vi "FormCalibra6.vi"() -> ()   [LabVIEW 2014]
uses:
  testMachine.ctl
  mainMachine.ctl
  <vilib>/Analysis/baseanly.llb/Mean (DBL).vi
  <vilib>/express/express shared/transition.llb/Dynamic To Waveform Array.vi
  <vilib>/express/express signal manip/GetorSetDDTAttributes/Set DDT Attributes/SetT0.vi
  <vilib>/express/express shared/transition.llb/Waveform Array To Dynamic.vi
  <vilib>/measure/mamon.llb/Trigger Detection for 1 Channel.vi
  <vilib>/express/express signal manip/GetorSetDDTAttributes/Set DDT Attributes/Set DDT Properties.xnode
  <vilib>/Analysis/NI_AALBase.lvlib
  <resource>/objmgr/daqmx.rc
  <vilib>/measure/NI_MAPro.lvlib
panel:
  in  "Lower level":dbl
  in  "hysteresis":dbl format="%.2p"
  in  "level":dbl format="%.2p"
  out "rpm":bool
  out "deviceName":tag
  out "editTotalWaitLimit":u8
  out "editCountWaitLimit":u8
  out "ledWaitState":bool caption="Wait State"
  out "sliderWaitUpperTime":u8(slide) max=50 scale=0.0..30.0
  out "slideWaitLowerTime":u8(slide) max=30 scale=0.0..1.0
  out "slideWaitTime":u8(slide) scale=0.0..150.0
  out "labelTestTime":string caption="Tempo total de ensaio"
  in  "buttonAcquisition":bool
  in  "editSetWaitTime":u8 caption="Tempo entre ciclos (s)" step=1 format="%0d"
  in  "stop":bool
  out "error out":errorcluster
  out "ledAcquireState":bool caption="Acquire State"
  out "editTotalLowerLimit":u8
  out "editCountLowerLimit":u8
  out "editTotalUpperLimit":u8
  out "editCountUpperLimit":u8
  out "ledEnsaio 3":bool
  out "ledBrakeState":bool caption="Brake State"
  out "ledExitState":bool caption="Exit State"
  out "ledMotorState":bool caption="Motor State"
  out "ledInit2State":bool caption="Init State"
  out "ledBlockState":bool caption="Block State"
  out "ledRunningState":bool caption="Running State"
  out "ledReadyState":bool caption="Ready State"
  out "ledInitState":bool caption="Init State"
  out "mainMachine":T1
  out "testMachine":T2=enum."finish"
  in  "editSetPathToFile":path
  in  "buttonStop":bool
  in  "buttonStart":bool
  out "graphForce":dynamicdata(graph)
  in  "editOffsetForce":dbl caption="Tara" min=0.0 max=100.0 step=0.1
  in  "editSetForce":dbl caption="Fator de conversão"
  out "editForce":dbl caption="Força (Kgf)" format="%#_4f"
  out "graphSpeed":dynamicdata(graph)
  in  "editSetSpeed":dbl caption="Fator de conversão"
  out "editSpeed":dbl caption="Velocidade (km/h)" format="%#_4f"
  out "editEngineSpeed":dbl caption="Rotação (RPM)" format="%#_4f"
  in  "buttonMotor":bool
  in  "buttonBrake":bool
  in  "editSetWaitLowerTime":u8 caption="Tempo de espera (s)"
  in  "editSetWaitUpperTime":u8=3 caption="Tempo de espera (s)"
  in  "editSetNumberOfCycles":u16 caption="Número de ciclos" max=999 step=1 format="%0d"
  in  "editSetLowerLimit":u32 caption="Limite inferior (km/h)"
  in  "editSetUpperLimit":u32 caption="Limite superior (km/h)"
  out "editTempB":dbl caption="Temperatura B (ºC)"
  out "editTempA":dbl caption="Temperatura A (ºC)"
  in  "editSetTempRef":dbl caption="Offset referência" step=0.01 format="%#_2f"
  out "editTempRef":dbl caption="Referência (ºC)"
  out "ledMotor":bool
  out "ledBrake":bool
  out "ledEnsaio":bool
  out "labelTotalCycle":string
  out "labelCurrentCycle":string
  out "labelSystemTitle":string
  in  "editCurrCycleCtr":u32
  in  "velocidade 2":u32
  out "velocidade":u32
  # "Bancada de Frenagem - Ensaio"
  # "Ensaio"
  # "Temperatura"
  # "Rotação"
  # "Célula de Carga"
  # "Configurações do ensaio"
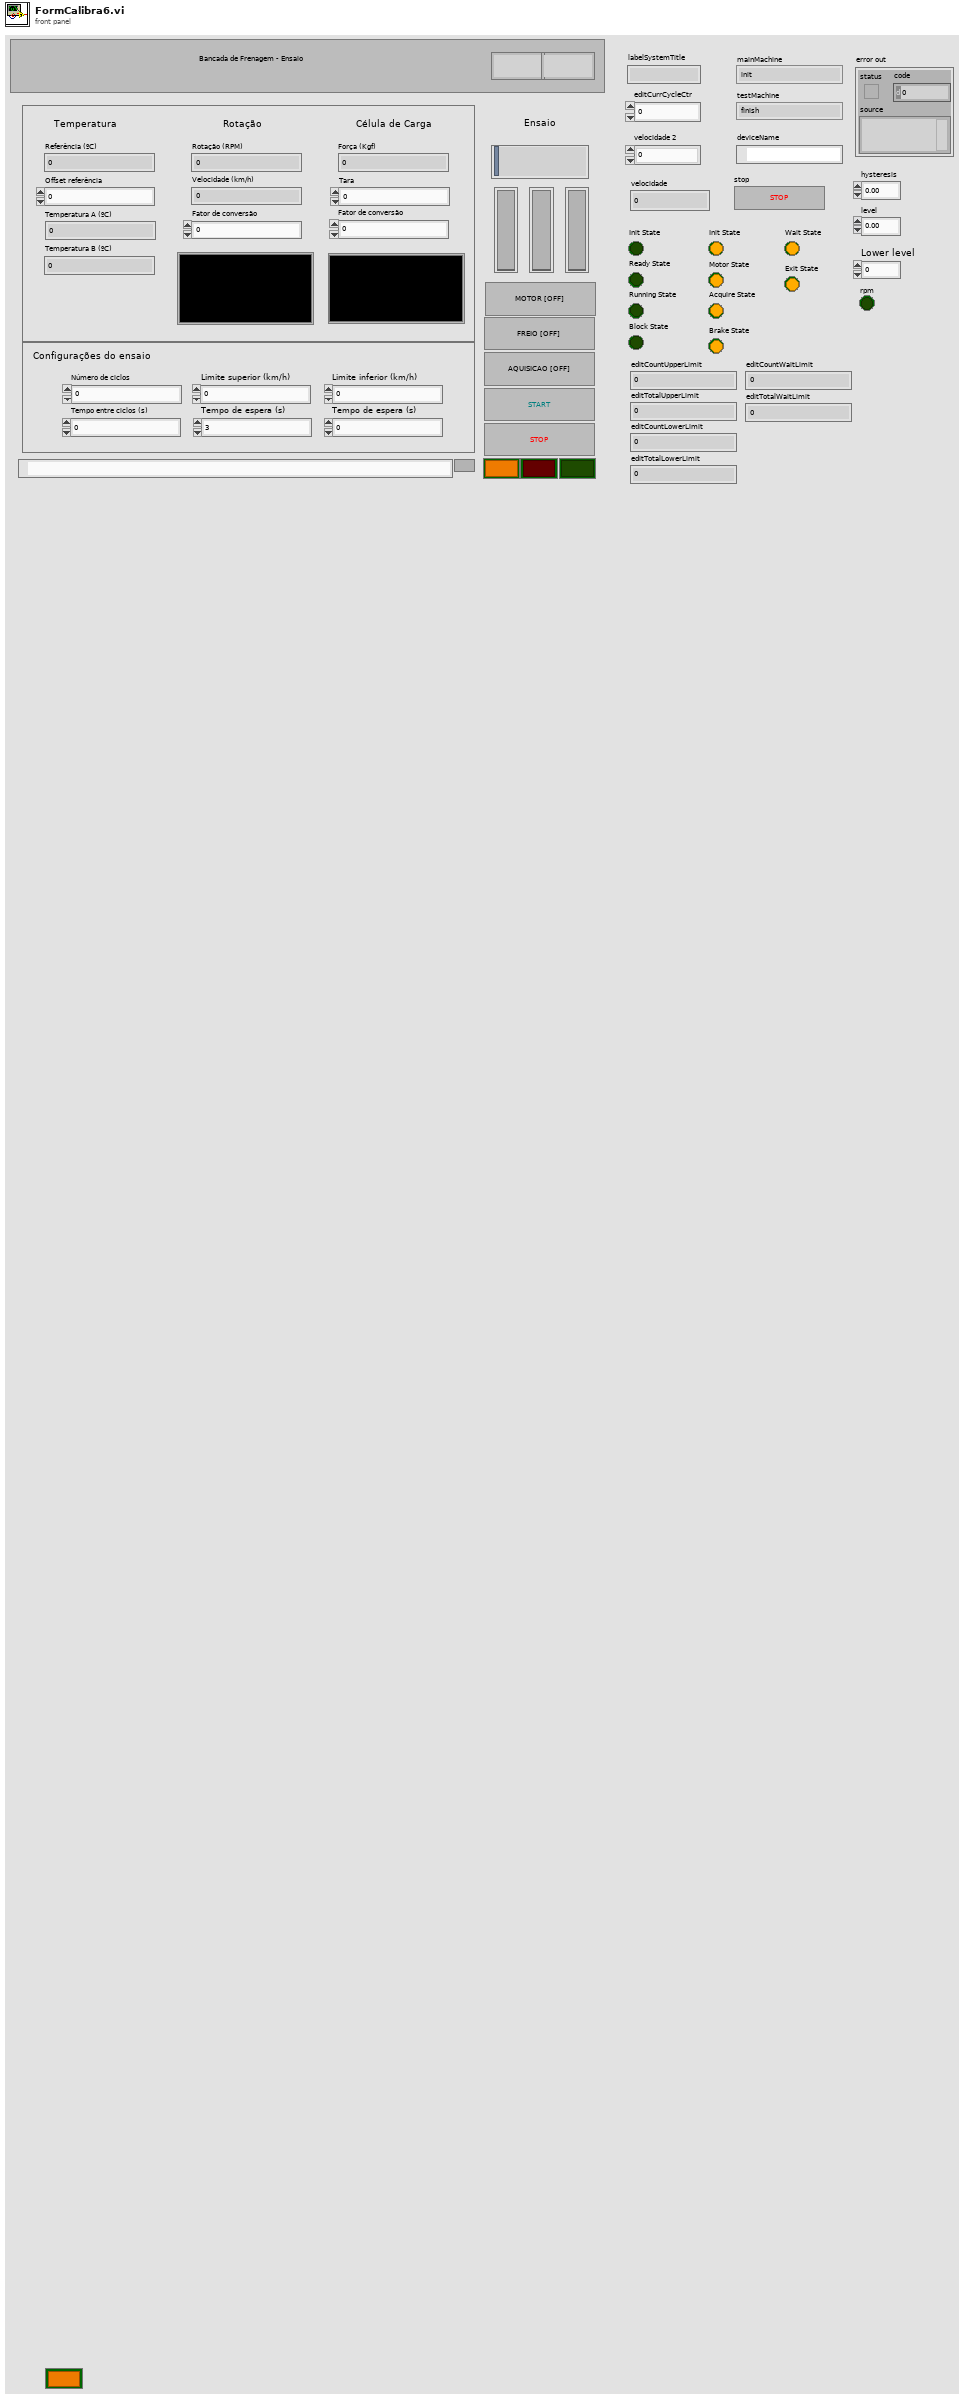
[diagram p1: front panel]
types:
  T1 = typedef "mainMachine.ctl" = enum16{"init", "ready", "running", "blocked", "finish"}
  T2 = typedef "testMachine.ctl" = enum16{"init", "motor", "motor acquire", "brake", "brake acquire", "wait ", "finish", "exit"}
  T3 = enum8{"Enabled", "Disabled", "Disabled and Grayed Out"}
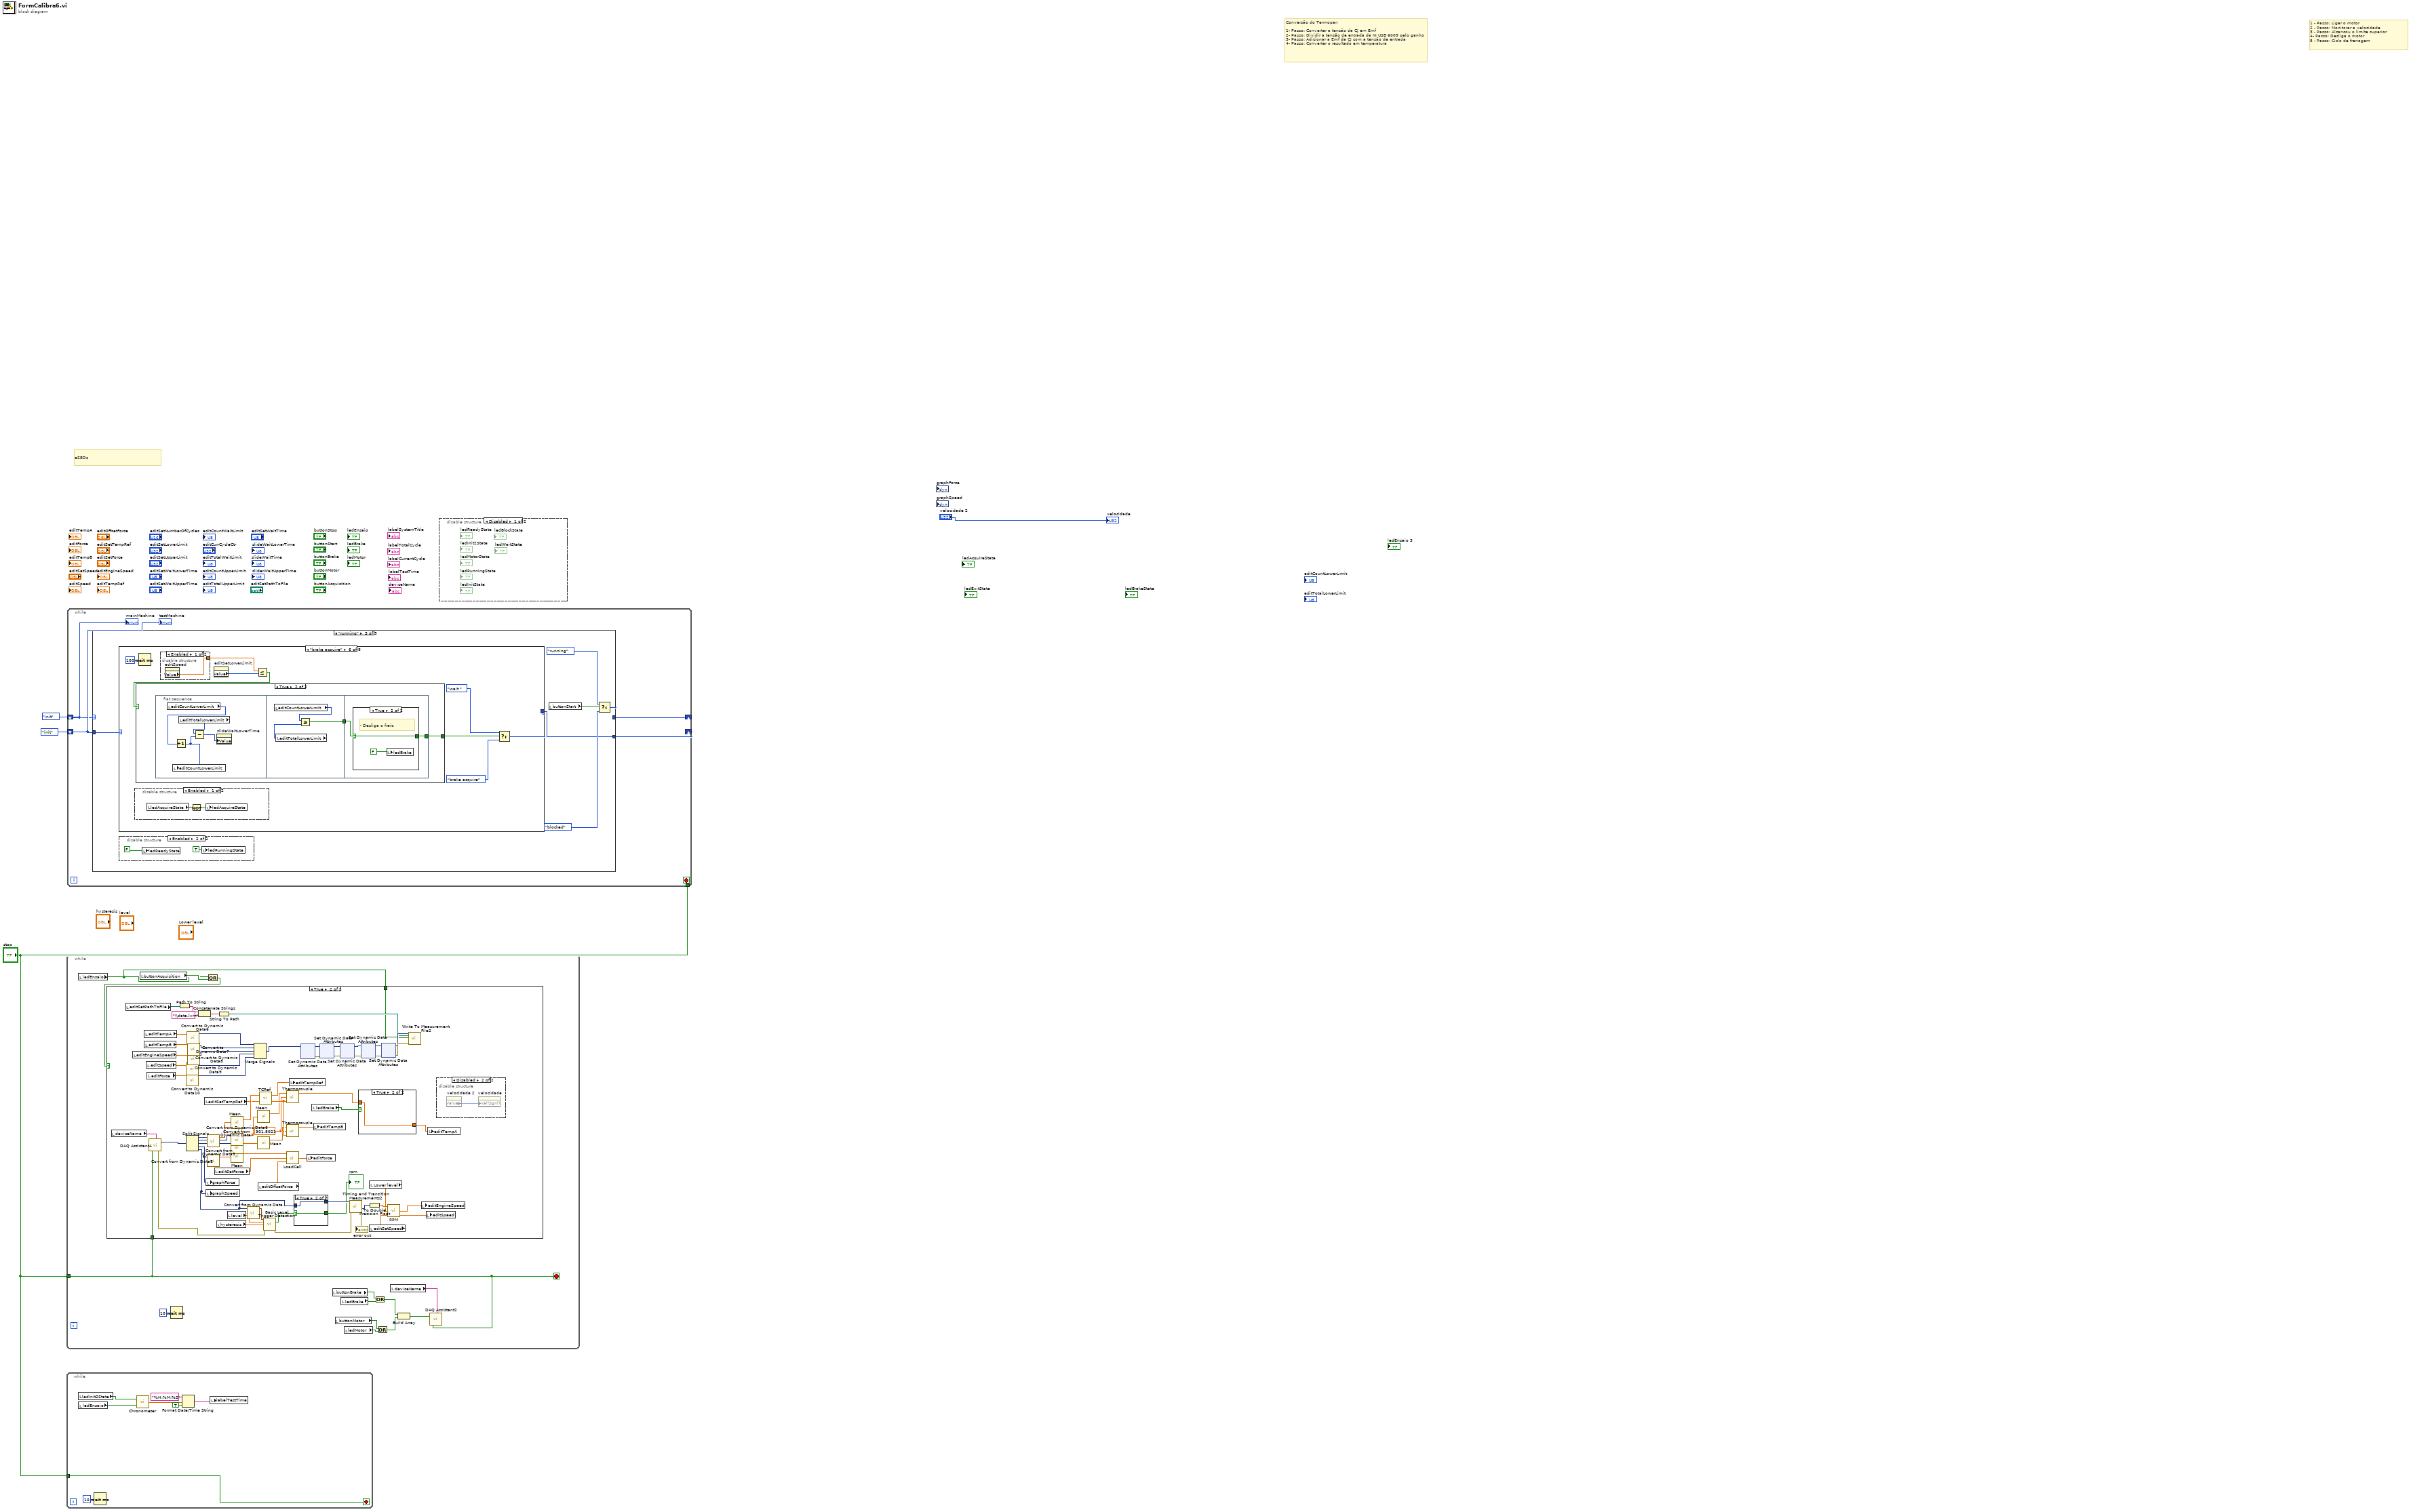
[diagram p0: block diagram]
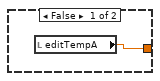
[diagram p4: hidden frame]
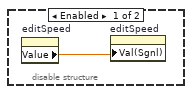
[diagram p6: hidden frame]
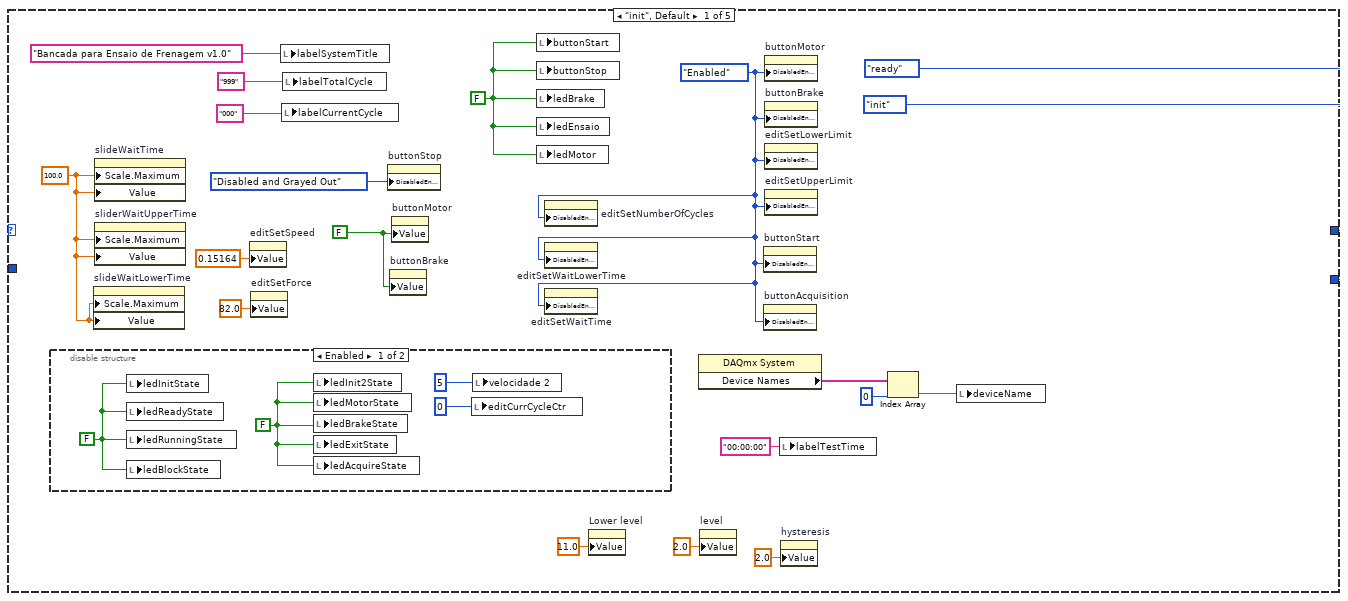
[diagram p7: hidden frame]
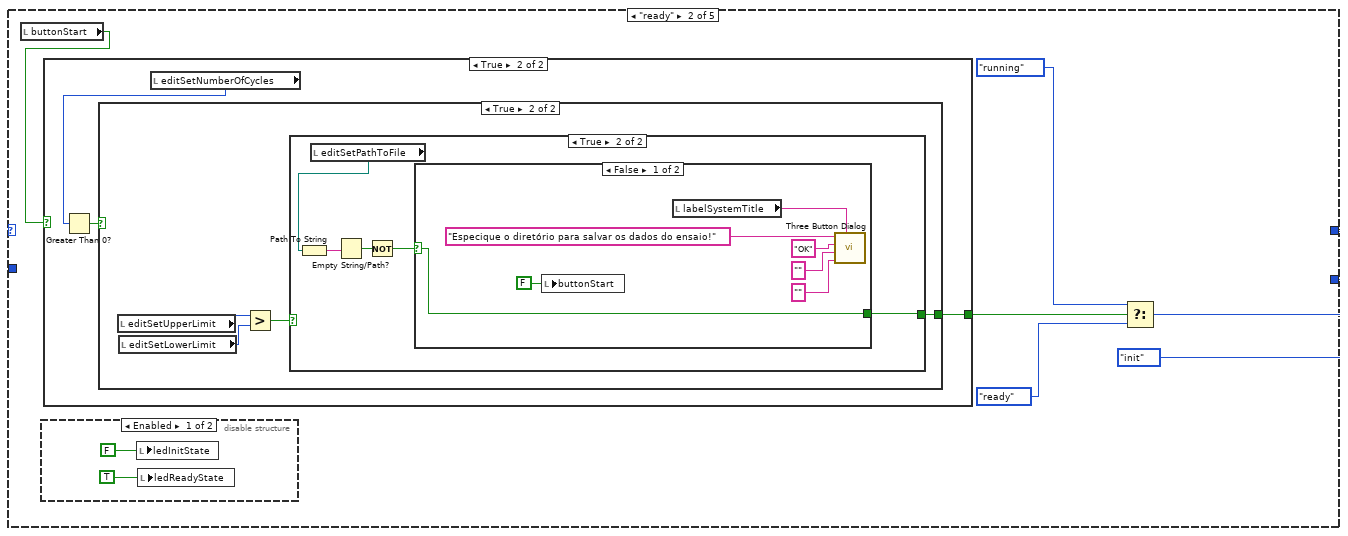
[diagram p9: hidden frame]
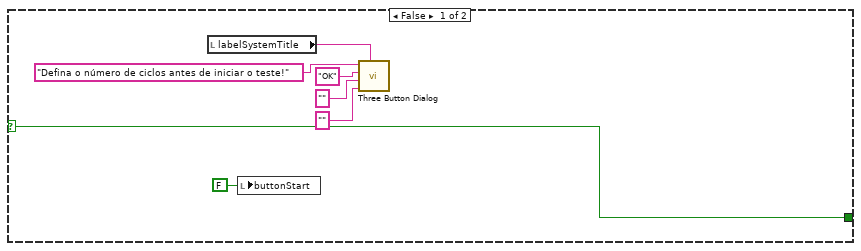
[diagram p12: hidden frame]
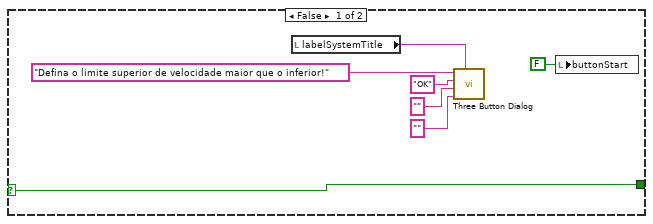
[diagram p13: hidden frame]
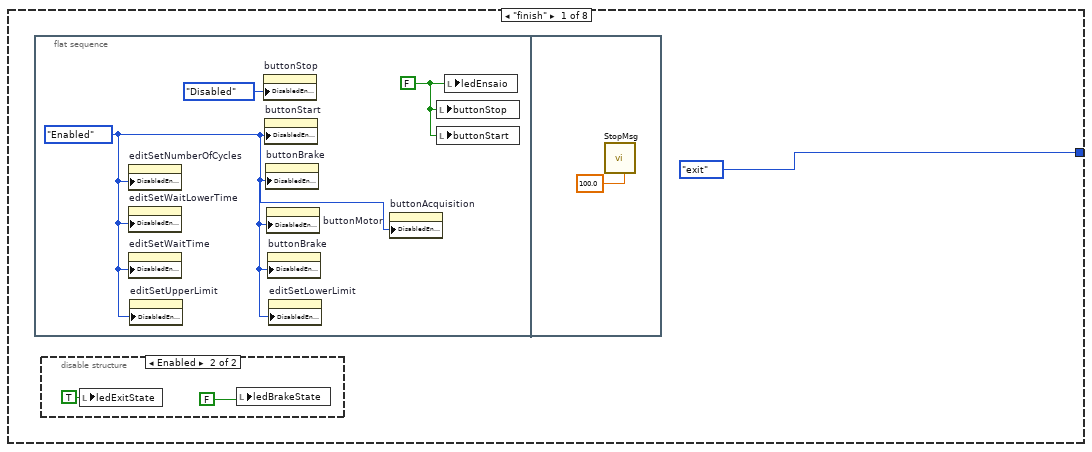
[diagram p16: hidden frame]
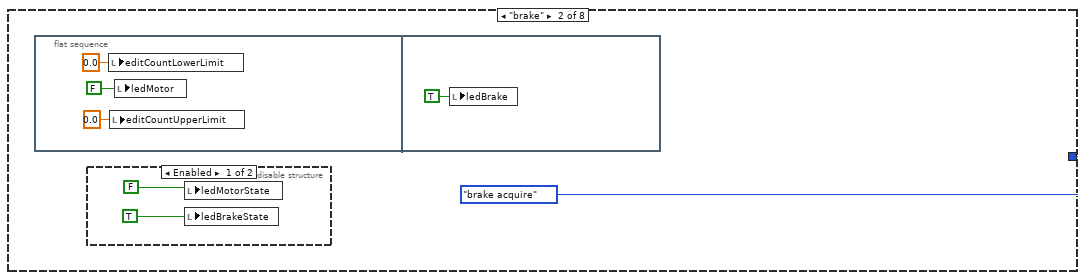
[diagram p18: hidden frame]
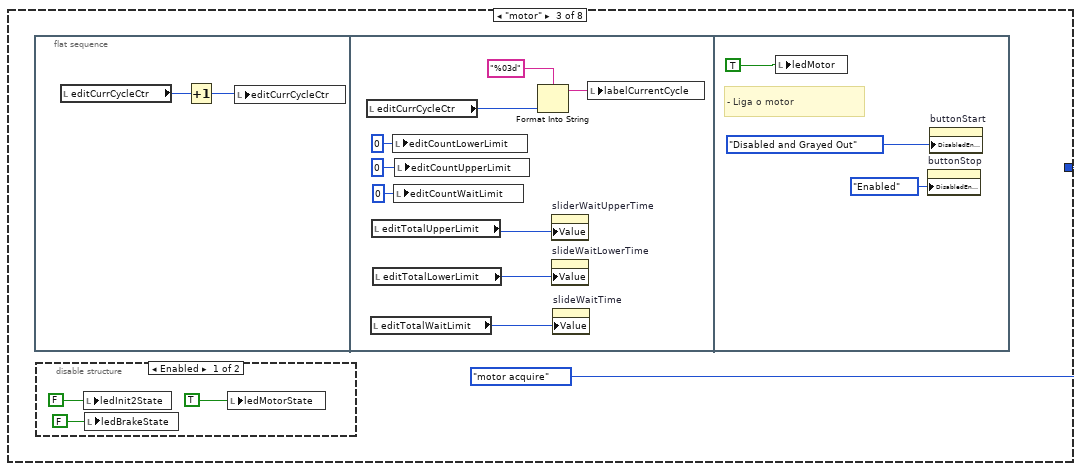
[diagram p20: hidden frame]
diagram:
  # "eSEDs"
  # "1 - Passo: Ligar o motor\n2 - Passo: Monitorar a velocidade\n3 - Passo: Alcancou o limite superior\n4- Passo: Desliga o motor\n5 - Passo: Ciclo de frenagem"
  # "Conversão do Termopar:\n\n1- Passo: Converter a tensão da CJ em Emf\n2- Passo: Dividir a tensão de entrada da NI USB 6009 pelo ganho\n3- Passo: Adicionar a Emf da CJ com a tensão de entrada\n4- Passo: Converter o resultado em temperatura"
  n1 = while {
    tunnel: "stop" -> [w12]
    stop <- w12 stop-if-true
    n2 = local read "ledInit2State"() -> (w6:bool)
    n3 = local read "ledEnsaio"() -> (w5:bool)
    n4 = Wait (ms)(milliseconds to wait=u32 10) -> ()  [unwired: 1 out]
    n5 = call "Chronometer.vi"("start"=w5, "reset"=w6) -> ("Time"=w10:dbl)
    n6 = Format Date/Time String(time format string (%c)="%H:%M:%S", seconds (now)=w10, UTC format=TRUE) -> (date/time string=w7:string)
    n7 = local write "labelTestTime"(w7) -> ()
  }
  n8 = while {
    tunnel: "stop" -> [w18]
    stop <- w18 stop-if-true
    n9 = local read "ledEnsaio"() -> (w15:bool)
    n10 = local read "buttonAcquisition"() -> (w17:bool)
    n11 = Wait (ms)(milliseconds to wait=u32 10) -> ()  [unwired: 1 out]
    n12 = Or(x=w15, y=w17) -> (x .or. y?=w16:bool)
    n13 = case shown="True" w16 {
      tunnel: w18 -> [_ w43]
      tunnel: w15 -> [_ w42]
      frame False {
      }
      frame True {
        w56 = 301.8021 ("factor")
        n14 = local read "deviceName"() -> (w41:tag)
        n15 = local read "editSetPathToFile"() -> (w70:path)
        n16 = local read "editEngineSpeed"() -> (w85:dbl)
        n17 = local read "editTempA"() -> (w82:dbl)
        n18 = local read "editTempB"() -> (w84:dbl)
        n19 = local read "editSpeed"() -> (w86:dbl)
        n20 = local read "editForce"() -> (w87:dbl)
        n21 = call "DAQ Assistant4"("stop (F)"=w43, "device name"=w41) -> ("data"=w45:dynamicdata, "error out"=w40:errorcluster)  [unwired: 14 in, 2 out]
        n22 = Path To String(path=w70) -> (string=w69:string)
        n23 = call "Convert to Dynamic Data9"("Double"=w86) -> ("Dynamic Data Type"=w90:dynamicdata)  [unwired: 3 in]
        n24 = call "Convert to Dynamic Data10"("Double"=w87) -> ("Dynamic Data Type"=w91:dynamicdata)  [unwired: 3 in]
        n25 = Split Signals(w45) -> (w48:dynamicdata, w52:dynamicdata, w50:dynamicdata, w60:dynamicdata, w37:dynamicdata)  [unwired: 5 in]
        n26 = call "Convert to Dynamic Data6"("Double"=w82) -> ("Dynamic Data Type"=w83:dynamicdata)  [unwired: 3 in]
        n27 = call "Convert to Dynamic Data7"("Double"=w84) -> ("Dynamic Data Type"=w88:dynamicdata)  [unwired: 3 in]
        n28 = call "Convert to Dynamic Data8"("Double"=w85) -> ("Dynamic Data Type"=w89:dynamicdata)  [unwired: 3 in]
        n29 = Concatenate Strings(w69, "\\data.lvm" ("string")) -> (w72:string)
        n30 = local read "editSetTempRef"() -> (w47:dbl)
        n31 = local write "graphForce"(w60) -> ()
        n32 = local write "graphSpeed"(w37) -> ()
        n33 = call "Convert from Dynamic Data5"("Dynamic Data Type"=w48) -> ("Array"=w67:dbl[])  [unwired: 3 in]
        n34 = call "Convert from Dynamic Data8"("Dynamic Data Type"=w60) -> ("Array"=w53:dbl[])  [unwired: 3 in]
        n35 = local read "editSetForce"() -> (w65:dbl)
        n36 = local read "hysteresis"() -> (w31:dbl)
        n37 = String To Path(string=w72) -> (path=w73:path)
        n38 = local read "level"() -> (w30:dbl)
        n39 = call-poly <vilib>:"Mean.vi"("X"=w67) -> ("mean"=w68:dbl)  [unwired: 1 out]
        n40 = call "Convert from Dynamic Data6"("Dynamic Data Type"=w52) -> ("Array"=w49:dbl[])  [unwired: 3 in]
        n41 = call "Convert from Dynamic Data7"("Dynamic Data Type"=w50) -> ("Array"=w51:dbl[])  [unwired: 3 in]
        n42 = call-poly <vilib>:"Mean.vi"("X"=w53) -> ("mean"=w59:dbl)  [unwired: 1 out]
        n43 = call "Convert from Dynamic Data"("Dynamic Data Type"=w37) -> ("Waveform"=w36:waveform(dbl))  [unwired: 3 in]
        n44 = Merge Signals(w83, w88, w89, w90, w91) -> (w92:dynamicdata)
        n45 = call-poly <vilib>:"Mean.vi"("X"=w49) -> ("mean"=w54:dbl)  [unwired: 1 out]
        n46 = call-poly <vilib>:"Mean.vi"("X"=w51) -> ("mean"=w55:dbl)  [unwired: 1 out]
        n47 = local read "editOffsetForce"() -> (w66:dbl)
        n48 = call "TCRef.vi"("offset"=w47, "data"=w68) -> ("emf(mV)"=w57:dbl, "temp (degC)"=w46:dbl)
        n49 = call-poly <vilib>:"Basic Level Trigger Detection.vi"("signal in"=w36, "level"=w30, "hysteresis"=w31, "error in (no error)"=w40) -> ("trigger detected?"=w35:bool, "error out"=w39:errorcluster)  [unwired: 9 in, 1 out]
        n50 = call "Thermocouple.vi"("cj(mV)"=w57, "factor"=w56, "data"=w54) -> ("temp(degC)"=w27:dbl)  [unwired: 2 out]
        n51 = call "Thermocouple.vi"("cj(mV)"=w57, "factor"=w56, "data"=w55) -> ("temp(degC)"=w58:dbl)  [unwired: 2 out]
        n52 = call "LoadCell.vi"("tara"=w66, "factor"=w65, "data"=w59) -> ("force (Kgf)"=w62:dbl)
        n53 = local write "editTempRef"(w46) -> ()
        n54 = case shown="True" w35 {
          selector: w35 -> [w97 w98]
          tunnel: w37 -> [_ w99]
          tunnel: [_ w99] -> w38
          tunnel: [w97 w98] -> w34
          frame False {
          }
          frame True {
          }
        }
        "rpm" <- w34
        n55 = xnode ("Set Dynamic Data Attributes")("Signals In"=w92) -> ("Signals Out"=w74:dynamicdata, "error out"=w76:errorcluster)  [unwired: 4 in]
        n56 = local write "editForce"(w62) -> ()
        n57 = local read "ledBrake"() -> (w28:bool)
        n58 = local write "editTempB"(w58) -> ()
        n59 = xnode ("Set Dynamic Data Attributes")("Signals In"=w74, "error in"=w76) -> ("Signals Out"=w75:dynamicdata, "error out"=w77:errorcluster)  [unwired: 3 in]
        n60 = xnode ("Set Dynamic Data Attributes")("Signals In"=w75, "error in"=w77) -> ("Signals Out"=w93:dynamicdata, "error out"=w78:errorcluster)  [unwired: 3 in]
        n61 = call "Timing and Transition Measurements2"("error in (no error)"=w39, "Signals"=w38) -> ("error out"=→"error out":errorcluster, "Frequency"=w33:dynamicdata)  [unwired: 8 in]
        n62 = case shown="True" w28 {
          tunnel: w27 -> [_ w96]
          tunnel: [w95 w96] -> w26
          frame False {
            n63 = local read "editTempA"() -> (w95:dbl)
          }
          frame True {
          }
        }
        n64 = xnode ("Set Dynamic Data Attributes")("Signals In"=w93, "error in"=w78) -> ("Signals Out"=w94:dynamicdata, "error out"=w79:errorcluster)  [unwired: 3 in]
        n65 = To Double Precision Float(number=w33) -> (double precision float=w32:dbl)
        n66 = local read "Lower level"() -> (w29:dbl)
        n67 = local read "editSetSpeed"() -> (w61:dbl)
        n68 = xnode ("Set Dynamic Data Attributes")("Signals In"=w94, "error in"=w79) -> ("Signals Out"=w80:dynamicdata, "error out"=w81:errorcluster)  [unwired: 3 in]
        n69 = call "RPM.vi"("factor"=w61, "Lower level"=w29, "data"=w32) -> ("km/h"=w64:dbl, "RPM"=w63:dbl)  [unwired: 1 out]
        n70 = call "Write To Measurement File2"("Signals"=w80, "Enable"=w42, "error in (no error)"=w81, "Filename"=w73) -> ()  [unwired: 13 in, 3 out]
        n71 = local write "editEngineSpeed"(w63) -> ()
        n72 = local write "editSpeed"(w64) -> ()
        n73 = local write "editTempA"(w26) -> ()
        n74 = disable-structure shown="Disabled" {
          frame Enabled {
            n75 = property on="editSpeed" class="DigNum (strict)"() -> ("Value"=w100:dbl)  [unwired: 2 in, 2 out]
            n76 = property on="editSpeed" class="DigNum (strict)"("Val(Sgnl)"=w100) -> ()  [unwired: 2 in, 2 out]
          }
          frame Disabled {
            n77 = property on="velocidade 2" class="DigNum (strict)"() -> ("Value"=w101:u32)  [unwired: 2 in, 2 out]
            n78 = property on="velocidade" class="DigNum (strict)"("Val(Sgnl)"=w101) -> ()  [unwired: 2 in, 2 out]
          }
        }
      }
    }
    n79 = local read "buttonBrake"() -> (w22:bool)
    n80 = local read "buttonMotor"() -> (w20:bool)
    n81 = local read "ledBrake"() -> (w24:bool)
    n82 = local read "ledMotor"() -> (w21:bool)
    n83 = Or(x=w22, y=w24) -> (x .or. y?=w23:bool)
    n84 = Or(x=w20, y=w21) -> (x .or. y?=w19:bool)
    n85 = local read "deviceName"() -> (w13:tag)
    n86 = Build Array(w23, w19) -> (w25:bool[])
    n87 = call "DAQ Assistant2"("data"=w25, "stop (T)"=w18, "device name"=w13) -> ()  [unwired: 15 in, 2 out]
  }
  n88 = while {
    shift-right: [w196] -> _
    shift-left: mainMachine."init" ("mainMachine") -> [w193]
    shift-right: [w195] -> _
    shift-left: testMachine."init" ("testMachine") -> [w194]
    tunnel: "stop" -> [w192]
    stop <- w192 stop-if-true
    n89 = case shown="\"running\"" w193 {
      tunnel: [mainMachine."ready" ("mainMachine") w220 w265 w405 mainMachine."finish" ("mainMachine")] -> w196
      tunnel: [testMachine."init" ("testMachine") testMachine."init" ("testMachine") w264 testMachine."init" ("testMachine") testMachine."init" ("testMachine")] -> w195
      tunnel: w194 -> [_ _ w263 _ _]
      frame "init", Default {
        w206 = 100.0 ("Scale.Range:Maximum")
        w207 = T3."Enabled" ("Disabled")
        w208 = FALSE ("buttonMotor")
        w214 = FALSE ("motor")
        n90 = disable-structure shown="Enabled" {
          frame Enabled {
            w216 = FALSE
            w217 = FALSE
            n91 = local write "ledInitState"(w217) -> ()
            n92 = local write "ledReadyState"(w217) -> ()
            n93 = local write "ledRunningState"(w217) -> ()
            n94 = local write "ledBlockState"(w217) -> ()
            n95 = local write "ledInit2State"(w216) -> ()
            n96 = local write "ledMotorState"(w216) -> ()
            n97 = local write "ledBrakeState"(w216) -> ()
            n98 = local write "ledExitState"(w216) -> ()
            n99 = local write "ledAcquireState"(w216) -> ()
            n100 = local write "editCurrCycleCtr"(u32 0 ("currentCycleCtr")) -> ()
            n101 = local write "velocidade 2"(u32 5 ("velocidade 2")) -> ()
          }
          frame Disabled {
          }
        }
        n102 = property on="slideWaitLowerTime" class="Slide (strict)"("Scale.Maximum"=w206, "Value"=w206) -> ()  [unwired: 2 in, 2 out]
        n103 = property on="slideWaitTime" class="Slide (strict)"("Scale.Maximum"=w206, "Value"=w206) -> ()  [unwired: 2 in, 2 out]
        n104 = property on="sliderWaitUpperTime" class="Slide (strict)"("Scale.Maximum"=w206, "Value"=w206) -> ()  [unwired: 2 in, 2 out]
        n105 = property on="editSetSpeed" class="DigNum (strict)"("Value"=0.15164 ("editSetSpeed")) -> ()  [unwired: 2 in, 2 out]
        n106 = property on="editSetForce" class="DigNum (strict)"("Value"=82.0 ("editSetForce")) -> ()  [unwired: 2 in, 2 out]
        n107 = local write "labelSystemTitle"("Bancada para Ensaio de Frenagem v1.0" ("systemTitle")) -> ()
        n108 = local write "labelCurrentCycle"("000" ("currentCycle")) -> ()
        n109 = local write "labelTotalCycle"("999" ("totalCycle")) -> ()
        n110 = property on="buttonStop" class="Bool (strict)"("DisabledEnum"=T3."Disabled and Grayed Out" ("Disabled")) -> ()  [unwired: 2 in, 2 out]
        n111 = property on="buttonBrake" class="Bool (strict)"("Value"=w208) -> ()  [unwired: 2 in, 2 out]
        n112 = property on="buttonMotor" class="Bool (strict)"("Value"=w208) -> ()  [unwired: 2 in, 2 out]
        n113 = local write "buttonStart"(w214) -> ()
        n114 = local write "buttonStop"(w214) -> ()
        n115 = local write "ledBrake"(w214) -> ()
        n116 = local write "ledEnsaio"(w214) -> ()
        n117 = local write "ledMotor"(w214) -> ()
        n118 = property on="editSetNumberOfCycles" class="DigNum (strict)"("DisabledEnum"=w207) -> ()  [unwired: 2 in, 2 out]
        n119 = property on="editSetWaitLowerTime" class="DigNum (strict)"("DisabledEnum"=w207) -> ()  [unwired: 2 in, 2 out]
        n120 = property on="editSetWaitTime" class="DigNum (strict)"("DisabledEnum"=w207) -> ()  [unwired: 2 in, 2 out]
        n121 = property on="Lower level" class="DigNum (strict)"("Value"=11.0 ("Lower level")) -> ()  [unwired: 2 in, 2 out]
        n122 = property class="DAQmx System"() -> ("Device Names"=w205:tag[])  [unwired: 2 in, 2 out]
        n123 = property on="level" class="DigNum (strict)"("Value"=2.0 ("level")) -> ()  [unwired: 2 in, 2 out]
        n124 = property on="buttonStart" class="Bool (strict)"("DisabledEnum"=w207) -> ()  [unwired: 2 in, 2 out]
        n125 = property on="buttonAcquisition" class="Bool (strict)"("DisabledEnum"=w207) -> ()  [unwired: 2 in, 2 out]
        n126 = property on="buttonMotor" class="Bool (strict)"("DisabledEnum"=w207) -> ()  [unwired: 2 in, 2 out]
        n127 = property on="buttonBrake" class="Bool (strict)"("DisabledEnum"=w207) -> ()  [unwired: 2 in, 2 out]
        n128 = property on="editSetLowerLimit" class="DigNum (strict)"("DisabledEnum"=w207) -> ()  [unwired: 2 in, 2 out]
        n129 = property on="editSetUpperLimit" class="DigNum (strict)"("DisabledEnum"=w207) -> ()  [unwired: 2 in, 2 out]
        n130 = local write "labelTestTime"("00:00:00" ("labelTestTime")) -> ()
        n131 = property on="hysteresis" class="DigNum (strict)"("Value"=2.0 ("hysteresis")) -> ()  [unwired: 2 in, 2 out]
        n132 = Index Array(array=w205, index=0) -> (element=w203:tag)
        n133 = local write "deviceName"(w203) -> ()
      }
      frame "ready" {
        n134 = local read "buttonStart"() -> (w223:bool)
        n135 = disable-structure shown="Enabled" {
          frame Enabled {
            n136 = local write "ledInitState"(FALSE ("ledReady")) -> ()
            n137 = local write "ledReadyState"(TRUE ("ledReady")) -> ()
          }
          frame Disabled {
          }
        }
        n138 = case shown="True" w223 {
          selector: w223 -> [w228 _]
          tunnel: [w228 w229] -> w222
          frame False {
          }
          frame True {
            n139 = local read "editSetNumberOfCycles"() -> (w230:u16)
            n140 = Greater Than 0?(x=w230) -> (x > 0?=w231:bool)
            n141 = case shown="True" w231 {
              selector: w231 -> [w238 _]
              tunnel: [w238 w239] -> w229
              frame False {
                n142 = local read "labelSystemTitle"() -> (w233:string)
                n143 = local write "buttonStart"(FALSE ("startButton")) -> ()
                n144 = call <vilib>:"Three Button Dialog.vi"("Window Title (\"\")"=w233, "Right Button Text (\"Cancel\")"="" ("Right Button Text (\"Cancel\")"), "Center Button Text (\"No\")"="" ("Center Button Text (\"No\")"), "Left Button Text (\"Yes\")"="OK" ("Left Button Text (\"Yes\")"), "message"="Defina o número de ciclos antes de iniciar o teste!") -> ()  [unwired: 6 in, 1 out]
              }
              frame True {
                n145 = local read "editSetUpperLimit"() -> (w241:u32)
                n146 = local read "editSetLowerLimit"() -> (w240:u32)
                n147 = Greater?(x=w241, y=w240) -> (0:w242:bool)
                n148 = case shown="True" w242 {
                  selector: w242 -> [w249 _]
                  tunnel: [w249 w252] -> w239
                  frame False {
                    n149 = local read "labelSystemTitle"() -> (w244:string)
                    n150 = call <vilib>:"Three Button Dialog.vi"("Window Title (\"\")"=w244, "Right Button Text (\"Cancel\")"="" ("Right Button Text (\"Cancel\")"), "Center Button Text (\"No\")"="" ("Center Button Text (\"No\")"), "Left Button Text (\"Yes\")"="OK" ("Left Button Text (\"Yes\")"), "message"="Defina o limite superior de velocidade maior que o inferior!") -> ()  [unwired: 6 in, 1 out]
                    n151 = local write "buttonStart"(FALSE ("startButton")) -> ()
                  }
                  frame True {
                    n152 = local read "editSetPathToFile"() -> (w254:path)
                    n153 = Path To String(path=w254) -> (string=w253:string)
                    n154 = Empty String/Path?(string/path=w253) -> (empty?=w251:bool)
                    n155 = Not(x=w251) -> (.not. x?=w250:bool)
                    n156 = case shown="False" w250 {
                      selector: w250 -> [w261 w262]
                      tunnel: [w261 w262] -> w252
                      frame False {
                        n157 = local write "buttonStart"(FALSE ("startButton")) -> ()
                        n158 = local read "labelSystemTitle"() -> (w256:string)
                        n159 = call <vilib>:"Three Button Dialog.vi"("Window Title (\"\")"=w256, "Right Button Text (\"Cancel\")"="" ("Right Button Text (\"Cancel\")"), "Center Button Text (\"No\")"="" ("Center Button Text (\"No\")"), "Left Button Text (\"Yes\")"="OK" ("Left Button Text (\"Yes\")"), "message"="Especique o diretório para salvar os dados do ensaio!") -> ()  [unwired: 6 in, 1 out]
                      }
                      frame True {
                      }
                    }
                  }
                }
              }
            }
          }
        }
        n160 = Select(t=mainMachine."running" ("mainMachine"), s=w222, f=mainMachine."ready" ("mainMachine")) -> (s? t:f=w220:T1)
      }
      frame "running" {
        n161 = case shown="\"brake acquire\"" w263 {
          tunnel: [testMachine."exit" ("testMachine") testMachine."brake acquire" ("testMachine") testMachine."motor acquire" ("testMachine") testMachine."motor" ("testMachine") w335 w355 testMachine."exit" ("testMachine") w388] -> w264
          frame "finish" {
            n162 = flat-sequence {
              frame #0 {
                w275 = FALSE ("ledReady")
                w274 = T3."Enabled" ("Disabled")
                n163 = property on="editSetNumberOfCycles" class="DigNum (strict)"("DisabledEnum"=w274) -> ()  [unwired: 2 in, 2 out]
                n164 = property on="editSetWaitLowerTime" class="DigNum (strict)"("DisabledEnum"=w274) -> ()  [unwired: 2 in, 2 out]
                n165 = property on="editSetWaitTime" class="DigNum (strict)"("DisabledEnum"=w274) -> ()  [unwired: 2 in, 2 out]
                n166 = property on="editSetUpperLimit" class="DigNum (strict)"("DisabledEnum"=w274) -> ()  [unwired: 2 in, 2 out]
                n167 = property on="buttonStop" class="Bool (strict)"("DisabledEnum"=T3."Disabled" ("Disabled")) -> ()  [unwired: 2 in, 2 out]
                n168 = property on="buttonStart" class="Bool (strict)"("DisabledEnum"=w274) -> ()  [unwired: 2 in, 2 out]
                n169 = property on="buttonBrake" class="Bool (strict)"("DisabledEnum"=w274) -> ()  [unwired: 2 in, 2 out]
                n170 = property on="buttonMotor" class="Bool (strict)"("DisabledEnum"=w274) -> ()  [unwired: 2 in, 2 out]
                n171 = property on="buttonBrake" class="Bool (strict)"("DisabledEnum"=w274) -> ()  [unwired: 2 in, 2 out]
                n172 = property on="editSetLowerLimit" class="DigNum (strict)"("DisabledEnum"=w274) -> ()  [unwired: 2 in, 2 out]
                n173 = property on="buttonAcquisition" class="Bool (strict)"("DisabledEnum"=w274) -> ()  [unwired: 2 in, 2 out]
                n174 = local write "buttonStop"(w275) -> ()
                n175 = local write "buttonStart"(w275) -> ()
                n176 = local write "ledEnsaio"(w275) -> ()
              }
              frame #1 {
                n177 = call "StopMsg.vi"("Max Value (100)"=100.0) -> ()  [unwired: 8 in, 2 out]
              }
            }
            n178 = disable-structure shown="Enabled" {
              frame Disabled {
              }
              frame Enabled {
                n179 = local write "ledExitState"(TRUE ("ledReady")) -> ()
                n180 = local write "ledBrakeState"(FALSE ("ledReady")) -> ()
              }
            }
          }
          frame "brake" {
            n181 = flat-sequence {
              frame #0 {
                n182 = local write "editCountLowerLimit"(0.0 ("editCountUpperLimit")) -> ()
                n183 = local write "editCountUpperLimit"(0.0 ("editCountUpperLimit")) -> ()
                n184 = local write "ledMotor"(FALSE ("motor")) -> ()
              }
              frame #1 {
                n185 = local write "ledBrake"(TRUE ("freio")) -> ()
              }
            }
            n186 = disable-structure shown="Enabled" {
              frame Enabled {
                n187 = local write "ledMotorState"(FALSE ("ledReady")) -> ()
                n188 = local write "ledBrakeState"(TRUE ("ledReady")) -> ()
              }
              frame Disabled {
              }
            }
          }
          frame "motor" {
            n189 = flat-sequence {
              frame #0 {
                n190 = local read "editCurrCycleCtr"() -> (w290:u32)
                n191 = Increment(x=w290) -> (x+1=w289:u32)
                n192 = local write "editCurrCycleCtr"(w289) -> ()
              }
              frame #1 {
                n193 = local read "editCurrCycleCtr"() -> (w297:u32)
                n194 = local read "editTotalWaitLimit"() -> (w291:u8)
                n195 = local read "editTotalUpperLimit"() -> (w293:u8)
                n196 = local read "editTotalLowerLimit"() -> (w292:u8)
                n197 = local write "editCountLowerLimit"(u8 0 ("editCountLowerLimit")) -> ()
                n198 = local write "editCountWaitLimit"(u8 0 ("editCountWaitLimit")) -> ()
                n199 = local write "editCountUpperLimit"(u8 0 ("editCountUpperLimit")) -> ()
                n200 = Format Into String(format string="%03d", w297) -> (resulting string=w298:string)  [unwired: 2 in, 1 out]
                n201 = property on="sliderWaitUpperTime" class="Slide (strict)"("Value"=w293) -> ()  [unwired: 2 in, 2 out]
                n202 = property on="slideWaitLowerTime" class="Slide (strict)"("Value"=w292) -> ()  [unwired: 2 in, 2 out]
                n203 = property on="slideWaitTime" class="Slide (strict)"("Value"=w291) -> ()  [unwired: 2 in, 2 out]
                n204 = local write "labelCurrentCycle"(w298) -> ()
              }
              frame #2 {
                # "- Liga o motor"
                n205 = local write "ledMotor"(TRUE ("motor")) -> ()
                n206 = property on="buttonStop" class="Bool (strict)"("DisabledEnum"=T3."Enabled" ("Disabled")) -> ()  [unwired: 2 in, 2 out]
                n207 = property on="buttonStart" class="Bool (strict)"("DisabledEnum"=T3."Disabled and Grayed Out" ("Disabled")) -> ()  [unwired: 2 in, 2 out]
              }
            }
            n208 = disable-structure shown="Enabled" {
              frame Enabled {
                n209 = local write "ledInit2State"(FALSE ("ledReady")) -> ()
                n210 = local write "ledBrakeState"(FALSE ("ledReady")) -> ()
                n211 = local write "ledMotorState"(TRUE ("ledReady")) -> ()
              }
              frame Disabled {
              }
            }
          }
          frame "init", Default {
            n212 = stacked-sequence {
              frame #0 {
                w310 = FALSE ("ensaio")
                n213 = property on="buttonBrake" class="Bool (strict)"("Value"=w310) -> ()  [unwired: 2 in, 2 out]
                n214 = local write "ledMotor"(w310) -> ()
                n215 = local write "ledBrake"(w310) -> ()
                n216 = property on="buttonMotor" class="Bool (strict)"("Value"=w310) -> ()  [unwired: 2 in, 2 out]
                n217 = local read "editSetNumberOfCycles"() -> (w317:u16)
                n218 = local read "editSetWaitLowerTime"() -> (w311:u8)
                n219 = local read "editSetWaitUpperTime"() -> (w314:u8)
                n220 = local read "editSetWaitTime"() -> (w305:u8)
                n221 = Multiply(x=w305, y=u32 10) -> (x*y=w306:u32)
                n222 = Multiply(x=w311, y=u32 10) -> (x*y=w309:u32)
                n223 = Format Into String(format string="%03d", w317) -> (resulting string=w318:string)  [unwired: 2 in, 1 out]
                n224 = Multiply(x=w314, y=u32 10) -> (x*y=w308:u32)
                n225 = local write "editTotalLowerLimit"(w309) -> ()
                n226 = local write "editTotalUpperLimit"(w308) -> ()
                n227 = local write "editTotalWaitLimit"(w306) -> ()
                n228 = local write "labelTotalCycle"(w318) -> ()
                n229 = local write "editCurrCycleCtr"(u32 0 ("currentCycleCtr")) -> ()
                n230 = local write "labelCurrentCycle"("000" ("currentCycle")) -> ()
              }
              frame #1 {
                w326 = T3."Disabled" ("Disabled")
                n231 = property on="editSetNumberOfCycles" class="DigNum (strict)"("DisabledEnum"=w326) -> ()  [unwired: 2 in, 2 out]
                n232 = property on="editSetWaitLowerTime" class="DigNum (strict)"("DisabledEnum"=w326) -> ()  [unwired: 2 in, 2 out]
                n233 = property on="editSetWaitTime" class="DigNum (strict)"("DisabledEnum"=w326) -> ()  [unwired: 2 in, 2 out]
                n234 = local read "editTotalUpperLimit"() -> (w329:u8)
                n235 = property on="sliderWaitUpperTime" class="Slide (strict)"("Scale.Maximum"=w329, "Scale.Minimum"=0.0 ("Scale.Range:Minimum"), "Scale.Increment"=1.0 ("Scale.Range:Increment"), "Value"=w329) -> ()  [unwired: 2 in, 2 out]
                n236 = property on="buttonAcquisition" class="Bool (strict)"("DisabledEnum"=w326) -> ()  [unwired: 2 in, 2 out]
                n237 = local read "editTotalLowerLimit"() -> (w323:u8)
                n238 = property on="slideWaitLowerTime" class="Slide (strict)"("Scale.Maximum"=w323, "Scale.Minimum"=0.0 ("Scale.Range:Minimum"), "Scale.Increment"=1.0 ("Scale.Range:Increment"), "Value"=w323) -> ()  [unwired: 2 in, 2 out]
                n239 = local read "editTotalWaitLimit"() -> (w320:u8)
                n240 = property on="slideWaitTime" class="Slide (strict)"("Scale.Maximum"=w320, "Scale.Minimum"=0.0 ("Scale.Range:Minimum"), "Scale.Increment"=1.0 ("Scale.Range:Increment"), "Value"=w320) -> ()  [unwired: 2 in, 2 out]
                n241 = call "StarMsg.vi"("Show"=TRUE, "Max Value (100)"=100.0) -> ()  [unwired: 7 in, 2 out]
                n242 = property on="buttonMotor" class="Bool (strict)"("DisabledEnum"=w326) -> ()  [unwired: 2 in, 2 out]
                n243 = property on="buttonBrake" class="Bool (strict)"("DisabledEnum"=w326) -> ()  [unwired: 2 in, 2 out]
                n244 = property on="editSetLowerLimit" class="DigNum (strict)"("DisabledEnum"=w326) -> ()  [unwired: 2 in, 2 out]
                n245 = property on="editSetUpperLimit" class="DigNum (strict)"("DisabledEnum"=w326) -> ()  [unwired: 2 in, 2 out]
              }
              frame #2 {
                n246 = local write "ledEnsaio"(TRUE ("ensaio")) -> ()
              }
            }
            n247 = disable-structure shown="Enabled" {
              frame Enabled {
                n248 = local write "ledInit2State"(TRUE ("ledReady")) -> ()
              }
              frame Disabled {
              }
            }
          }
          frame "motor acquire" {
            n249 = disable-structure shown="Enabled" {
              frame Enabled {
                n250 = local read "ledAcquireState"() -> (w344:bool)
                n251 = Not(x=w344) -> (.not. x?=w343:bool)
                n252 = local write "ledAcquireState"(w343) -> ()
              }
              frame Disabled {
              }
            }
            n253 = Wait (ms)(milliseconds to wait=u32 100) -> ()  [unwired: 1 out]
            n254 = disable-structure shown="Enabled" {
              disable-tunnel: [w341 w342] -> w334
              frame Enabled {
                n255 = property on="editSpeed" class="DigNum (strict)"() -> ("Value"=w341:dbl)  [unwired: 2 in, 2 out]
              }
              frame Disabled {
                n256 = property on="velocidade" class="DigNum (strict)"() -> ("Value"=w342:u32)  [unwired: 2 in, 2 out]
              }
            }
            n257 = property on="editSetUpperLimit" class="DigNum (strict)"() -> ("Value"=w333:u32)  [unwired: 2 in, 2 out]
            n258 = Greater Or Equal?(x=w334, y=w333) -> (x >= y?=w339:bool)
            n259 = case shown="True" w339 {
              selector: w339 -> [w345 _]
              tunnel: [w345 w346] -> w338
              frame False {
              }
              frame True {
                n260 = flat-sequence {
                  tunnel: [w351] -> w346
                  frame #0 {
                    n261 = local read "editCountUpperLimit"() -> (w349:u8)
                    n262 = Increment(x=w349) -> (x+1=w347:u8)
                    n263 = local write "editCountUpperLimit"(w347) -> ()
                    n264 = local read "editTotalUpperLimit"() -> (w348:u8)
                    n265 = Subtract(x=w348, y=w347) -> (x-y=w350:u8)
                    n266 = property on="sliderWaitUpperTime" class="Slide (strict)"("Value"=w350) -> ()  [unwired: 2 in, 2 out]
                  }
                  frame #1 {
                    n267 = local read "editCountUpperLimit"() -> (w353:u8)
                    n268 = local read "editTotalUpperLimit"() -> (w352:u8)
                    n269 = Greater Or Equal?(x=w353, y=w352) -> (x >= y?=w351:bool)
                  }
                }
              }
            }
            n270 = Select(t=testMachine."brake" ("testMachine"), s=w338, f=testMachine."motor acquire" ("testMachine")) -> (s? t:f=w335:T2)
          }
          frame "brake acquire" {
            n271 = disable-structure shown="Enabled" {
              frame Enabled {
                n272 = local read "ledAcquireState"() -> (w363:bool)
                n273 = Not(x=w363) -> (.not. x?=w362:bool)
                n274 = local write "ledAcquireState"(w362) -> ()
              }
              frame Disabled {
              }
            }
            n275 = Wait (ms)(milliseconds to wait=u32 100) -> ()  [unwired: 1 out]
            n276 = disable-structure shown="Enabled" {
              disable-tunnel: [w364 w365] -> w354
              frame Enabled {
                n277 = property on="editSpeed" class="DigNum (strict)"() -> ("Value"=w364:dbl)  [unwired: 2 in, 2 out]
              }
              frame Disabled {
                n278 = property on="velocidade" class="DigNum (strict)"() -> ("Value"=w365:u32)  [unwired: 2 in, 2 out]
              }
            }
            n279 = property on="editSetLowerLimit" class="DigNum (strict)"() -> ("Value"=w356:u32)  [unwired: 2 in, 2 out]
            n280 = Less Or Equal?(x=w354, y=w356) -> (x <= y?=w360:bool)
            n281 = case shown="True" w360 {
              selector: w360 -> [w366 _]
              tunnel: [w366 w367] -> w358
              frame False {
              }
              frame True {
                n282 = flat-sequence {
                  tunnel: [w373] -> w368
                  tunnel: w368 -> [w377]
                  tunnel: [w376] -> w367
                  frame #0 {
                    n283 = local read "editCountLowerLimit"() -> (w372:u8)
                    n284 = Increment(x=w372) -> (x+1=w371:u8)
                    n285 = local write "editCountLowerLimit"(w371) -> ()
                    n286 = local read "editTotalLowerLimit"() -> (w370:u8)
                    n287 = Subtract(x=w370, y=w371) -> (x-y=w369:u8)
                    n288 = property on="slideWaitLowerTime" class="Slide (strict)"("Value"=w369) -> ()  [unwired: 2 in, 2 out]
                  }
                  frame #1 {
                    n289 = local read "editCountLowerLimit"() -> (w375:u8)
                    n290 = local read "editTotalLowerLimit"() -> (w374:u8)
                    n291 = Greater Or Equal?(x=w375, y=w374) -> (x >= y?=w373:bool)
                  }
                  frame #2 {
                    n292 = case shown="True" w377 {
                      selector: w377 -> [w378 w379]
                      tunnel: [w378 w379] -> w376
                      frame False {
                      }
                      frame True {
                        # "- Desliga o freio"
                        n293 = local write "ledBrake"(FALSE ("freio")) -> ()
                      }
                    }
                  }
                }
              }
            }
            n294 = Select(t=testMachine."wait " ("testMachine"), s=w358, f=testMachine."brake acquire" ("testMachine")) -> (s? t:f=w355:T2)
          }
          frame "exit" {
          }
          frame "wait " {
            # "- Aguarda 0.5s \n- Atualiza o numero de ciclos"
            n295 = flat-sequence {
              tunnel: [w394] -> w382
              frame #0 {
                n296 = local read "editCountWaitLimit"() -> (w390:u8)
                n297 = Increment(x=w390) -> (x+1=w391:u8)
                n298 = local write "editCountWaitLimit"(w391) -> ()
                n299 = local read "editTotalWaitLimit"() -> (w393:u8)
                n300 = Subtract(x=w393, y=w391) -> (x-y=w392:u8)
                n301 = property on="slideWaitTime" class="Slide (strict)"("Value"=w392) -> ()  [unwired: 2 in, 2 out]
              }
              frame #1 {
                n302 = local read "editCountWaitLimit"() -> (w396:u8)
                n303 = local read "editTotalWaitLimit"() -> (w395:u8)
                n304 = Greater Or Equal?(x=w396, y=w395) -> (x >= y?=w394:bool)
              }
            }
            n305 = disable-structure shown="Enabled" {
              frame Enabled {
                n306 = local read "ledWaitState"() -> (w403:bool)
                n307 = Not(x=w403) -> (.not. x?=w402:bool)
                n308 = local write "ledBrakeState"(FALSE ("ledBrakeState")) -> ()
                n309 = local write "ledWaitState"(w402) -> ()
              }
              frame Disabled {
              }
            }
            n310 = Wait (ms)(milliseconds to wait=u32 100) -> ()  [unwired: 1 out]
            n311 = case shown="True" w382 {
              selector: w382 -> [w397 _]
              tunnel: [w397 w401] -> w383
              frame False {
              }
              frame True {
                n312 = local read "editSetNumberOfCycles"() -> (w399:u16)
                n313 = local read "editCurrCycleCtr"() -> (w398:u32)
                n314 = Greater Or Equal?(x=w398, y=w399) -> (x >= y?=w401:bool)
                n315 = Not(x=w401) -> (.not. x?=w400:bool)
                n316 = local write "ledEnsaio"(w400) -> ()
              }
            }
            n317 = Select(t=testMachine."motor" ("testMachine"), s=w382, f=testMachine."wait " ("testMachine")) -> (s? t:f=w384:T2)
            n318 = Select(t=testMachine."finish" ("testMachine"), s=w383, f=w384) -> (s? t:f=w388:T2)
          }
        }
        n319 = disable-structure shown="Enabled" {
          frame Disabled {
          }
          frame Enabled {
            n320 = local write "ledReadyState"(FALSE ("ledReady")) -> ()
            n321 = local write "ledRunningState"(TRUE ("ledReady")) -> ()
          }
        }
        n322 = local read "buttonStart"() -> (w268:bool)
        n323 = Select(t=mainMachine."running" ("mainMachine"), s=w268, f=mainMachine."blocked" ("mainMachine")) -> (s? t:f=w265:T1)
      }
      frame "blocked" {
        n324 = local read "buttonStart"() -> (w409:bool)
        n325 = Select(t=mainMachine."ready" ("mainMachine"), s=w409, f=mainMachine."blocked" ("mainMachine")) -> (s? t:f=w405:T1)
        n326 = local write "ledRunningState"(FALSE ("ledReady")) -> ()
        n327 = local write "ledBlockState"(TRUE ("ledReady")) -> ()
      }
      frame "finish" {
        n328 = local write "ledBlockState"(FALSE ("ledReady")) -> ()
      }
    }
    "mainMachine" <- w193
    "testMachine" <- w194
  }
  n329 = disable-structure shown="Disabled" {
    frame Disabled {
    }
    frame Enabled {
    }
  }
  "velocidade" <- "velocidade 2"
